vi "Read Data Acquisition Memory.vi"(0 "VISA resource name":refnum<visa-resource-name>, 5 "Maximum Data Points (0)":i32 min=0 max=100 step=1, 11 "error in (no error)":errorcluster) -> (4 "VISA resource name out":refnum<visa-resource-name>, 6 "Data Acquisition":dbl[][](array[numeric]) format="%^#_6g", 8 "Read Data Points":i32, 10 "Available Data Points":i32, 15 "error out":errorcluster)   [LabVIEW 2017, in "HH PLI Series.lvlib"]
doc: "Reads stored data which has been acquired previously.\n\n<b>Note</b>\nSet Maximum data points to zero to get saved data points without reading data points.\nThe stored data may be read only when data acquisition is stopped."
uses:
  HH PLI Series.lvlib
panel:
  # "Timestamp [s]"
  # "Voltage [V]"
  # "Current [A]"
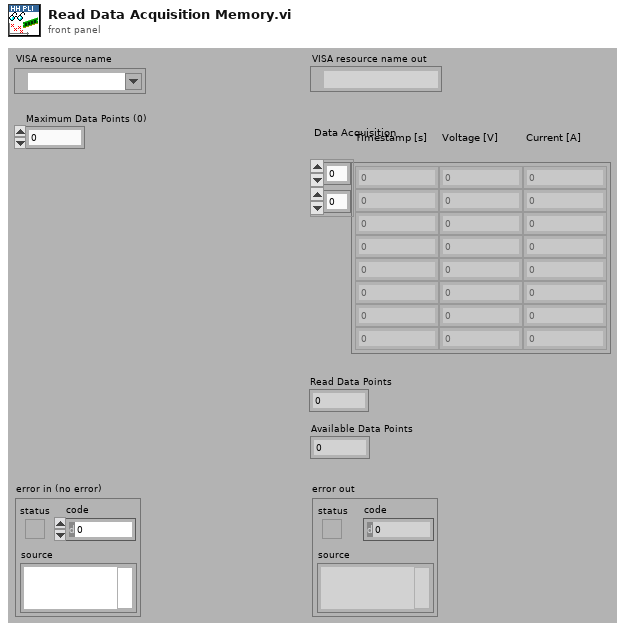
[diagram p1: front panel]
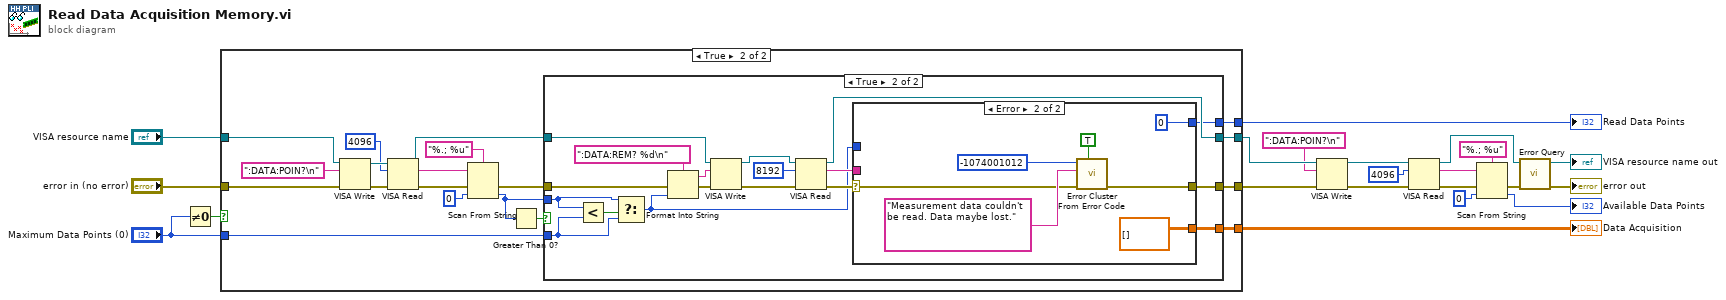
[diagram p0: block diagram]
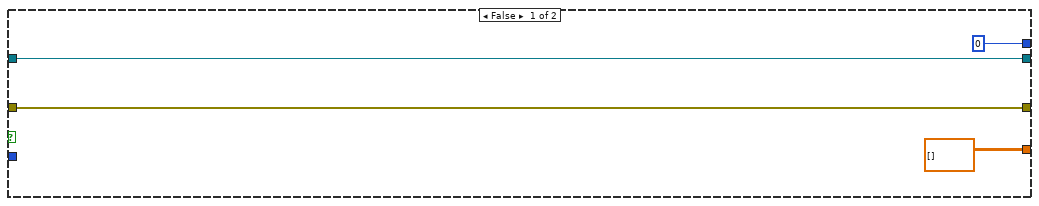
[diagram p2: hidden frame]
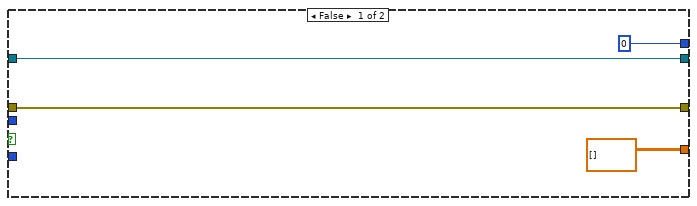
[diagram p3: hidden frame]
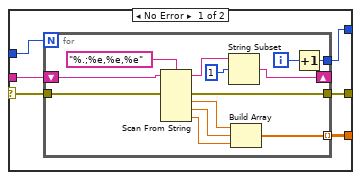
[diagram p4: hidden frame]
diagram:
  n1 = Not Equal To 0?(x="Maximum Data Points (0)") -> (x != 0?=w3:bool)
  n2 = case shown="True" w3 {
    tunnel: "VISA resource name" -> [w22 w44]
    tunnel: "error in (no error)" -> [w25 w43]
    tunnel: [dbl[][] [] w33] -> w17
    tunnel: "Maximum Data Points (0)" -> [_ w32]
    tunnel: [0 ("Maximum Data Points (0)") w30] -> w15
    tunnel: [w22 w29] -> w14
    tunnel: [w25 w28] -> w2
    frame False {
    }
    frame True {
      n3 = VISA Write(VISA resource name=w44, write buffer=":DATA:POIN?\n" ("initial string"), error in (no error)=w43) -> (VISA resource name out=w42:refnum<visa-resource-name>, error out=w41:errorcluster)  [unwired: 1 out]
      n4 = VISA Read(VISA resource name=w42, byte count=u32 4096, error in (no error)=w41) -> (VISA resource name out=w34:refnum<visa-resource-name>, read buffer=w36:string, error out=w37:errorcluster)  [unwired: 1 out]
      n5 = Scan From String(format string="%.; %u", input string=w36, error in=w37, default 1=0 ("default value 1")) -> (error out=w35:errorcluster, output 1=w31:i32)  [unwired: 1 in, 2 out]
      n6 = Greater Than 0?(x=w31) -> (x > 0?=w27:bool)
      n7 = case shown="True" w27 {
        tunnel: w32 -> [_ w61]
        tunnel: w35 -> [w46 w64]
        tunnel: w34 -> [w47 w53]
        tunnel: w31 -> [_ w62]
        tunnel: [dbl[][] [] w59] -> w33
        tunnel: [w46 w58] -> w28
        tunnel: [w47 w57] -> w29
        tunnel: [0 ("Maximum Data Points (0)") w49] -> w30
        frame False {
        }
        frame True {
          n8 = Less?(x=w62, y=w61) -> (x < y?=w63:bool)
          n9 = Select(t=w62, s=w63, f=w61) -> (s? t:f=w50:i32)
          n10 = Format Into String(format string=":DATA:REM? %d\n" ("initial string"), error in=w64, w50) -> (resulting string=w52:string, error out=w56:errorcluster)  [unwired: 1 in]
          n11 = VISA Write(VISA resource name=w53, write buffer=w52, error in (no error)=w56) -> (VISA resource name out=w54:refnum<visa-resource-name>, error out=w55:errorcluster)  [unwired: 1 out]
          n12 = VISA Read(VISA resource name=w54, byte count=u32 8192, error in (no error)=w55) -> (VISA resource name out=w57:refnum<visa-resource-name>, read buffer=w60:string, error out=w51:errorcluster)  [unwired: 1 out]
          n13 = case shown="Error" w51 {
            selector: w51 -> [w69 w87]
            tunnel: w60 -> [w72 _]
            tunnel: [w71 dbl[][] []] -> w59
            tunnel: [w70 w86] -> w58
            tunnel: w50 -> [w68 _]
            tunnel: [w67 0 ("Maximum Data Points (0)")] -> w49
            frame No Error {
              n14 = for {
                N: w68 -> [_]
                shift-right: [w78] -> _
                shift-left: w72 -> [w79]
                tunnel: w69 -> [w77]
                tunnel: [w76] -> w70
                tunnel: [w75] -> w71 mode=indexing
                tunnel: [w74] -> w67
                i -> [w73]
                n15 = Scan From String(format string="%.;%e,%e,%e", input string=w79, error in=w77) -> (remaining string=w84:string, error out=w76:errorcluster, output 1=w81:dbl, output 2=w82:dbl, output 3=w83:dbl)  [unwired: 4 in, 1 out]
                n16 = String Subset(string=w84, offset (0)=1) -> (substring=w78:string)  [unwired: 1 in]
                n17 = Build Array(w81, w82, w83) -> (w75:dbl[])
                n18 = Increment(x=w73) -> (x+1=w74:i32)
              }
            }
            frame Error {
              n19 = call <vilib>:"Error Cluster From Error Code.vi"("show call chain? (False)"=TRUE, "error in (no error)"=w87, "error message (\"\")"="Measurement data couldn't be read. Data maybe lost." ("error message (\"\")"), "error code (0)"=-1074001012) -> ("error out"=w86:errorcluster)  [unwired: 5 in]
            }
          }
        }
      }
    }
  }
  "Data Acquisition" <- w17
  "Read Data Points" <- w15
  n20 = VISA Write(VISA resource name=w14, write buffer=":DATA:POIN?\n" ("initial string"), error in (no error)=w2) -> (VISA resource name out=w7:refnum<visa-resource-name>, error out=w9:errorcluster)  [unwired: 1 out]
  n21 = VISA Read(VISA resource name=w7, byte count=u32 4096, error in (no error)=w9) -> (VISA resource name out=w6:refnum<visa-resource-name>, read buffer=w5:string, error out=w8:errorcluster)  [unwired: 1 out]
  n22 = Scan From String(format string="%.; %u", input string=w5, error in=w8, default 1=0 ("default value 1")) -> (error out=w11:errorcluster, output 1=→"Available Data Points":i32)  [unwired: 1 in, 2 out]
  n23 = call "Error Query.vi"("error in (no error)"=w11, "VISA resource name"=w6) -> ("error out"=→"error out":errorcluster, "VISA resource name out"=→"VISA resource name out":refnum<visa-resource-name>)  [unwired: 6 in, 2 out]
